vi "Filter Packets.vi"(7 "Offset in":i32, 10 "L2 Packet in":u8[](array[numeric]), 11 "L2Enet_RW_CORE":refnum<class "L2ENET_RW_CORE.lvclass">) -> (2 "Valid":bool)   [LabVIEW 2021, in "L2ENET_RW_CORE.lvclass"]
uses:
  L2ENET_RW_CORE.lvclass
  L2ENET_RW_CORE.lvclass/L2ENET_RW_CORE.ctl
  <vilib>/CIF Foundation/CIF Enet Parse and Build/Ethernet_Parse_Build_CIF.lvlib
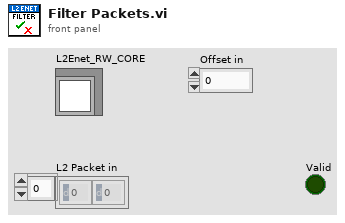
[diagram p1: front panel]
types:
  T1 = typedef "Ethernet_Parse_Build_CIF.lvlib/Filter.ctl" = cluster{"L2 Filter":T2, "IPV4 Filter":T3}
  T2 = typedef "Ethernet_Parse_Build_CIF.lvlib/L2 Filter.ctl" = cluster{"DMAC Filter":bool, "DMAC":u8[], "SMAC Filter":bool, "SMAC":u8[], "EtherType Filter":bool, "EtherType":u16, "VLAN Filter":bool, "VLAN":u16, "PCP Filter":bool, "PCP":u8}
  T3 = typedef "Ethernet_Parse_Build_CIF.lvlib/IPV4 Filter.ctl" = cluster{"Source IP Filter":bool, "Source IP Address":u32, "Destination  IP Filter":bool, "Dest IP Address":u32, "IP Protocol Filter":bool, "Protocol":T4, "Source Port Filter":bool, "Source Port":u16, "Dest Port Filter ":bool, "Dest Port":u16}
  T4 = typedef "Ethernet_Parse_Build_CIF.lvlib/IPV4 Protocol Ring.ctl" = u8
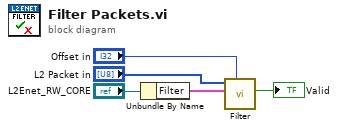
[diagram p0: block diagram]
diagram:
  n1 = Unbundle By Name("L2Enet_RW_CORE") -> ("Filter"=w4:T1[])
  n2 = call <vilib>:"Filter.vi"("Offset in"="Offset in", "Input Filter"=w4, "Raw Frame"="L2 Packet in") -> ("Pass Filter"=→"Valid":bool)  [unwired: 8 in]
